vi "RT Main.vi"() -> ()   [LabVIEW 2021]
doc: "Demonstrates the use of the UDP functions to receive broadcast data over a UDP connection."
uses:
  <vilib>/myRIO/Express VI/Onboard Devices/LED/LED Express VI.xnode
  <vilib>/myRIO/Instrument Drivers/Onboard IO/DIO/vis/Write.vi
  <vilib>/myRIO/Instrument Drivers/Onboard IO/DIO/DIO.lvlib
  <vilib>/myRIO/Common/Instrument Driver Framework/myRIO v1.0/DIO/typedefs/DIO Channels Enum.ctl
  <vilib>/myRIO/Common/Instrument Driver Framework/myRIO v1.0/DIO/typedefs/DIO Channels List.ctl
  <vilib>/myRIO/Common/Instrument Driver Framework/Utilities/typedefs/Generic FPGA Reference.ctl
  <vilib>/myRIO/Common/Instrument Driver Framework/Utilities/typedefs/myRIO v1.0 Reference.ctl
  <vilib>/myRIO/Common/Instrument Driver Framework/Utilities/typedefs/Hardware Version Enum.ctl
  <vilib>/myRIO/Common/Instrument Driver Framework/Utilities/typedefs/myRIO Generic Hardware Reference.ctl
  <vilib>/myRIO/Instrument Drivers/Onboard IO/DIO/typedefs/DIO Reference.ctl
  <vilib>/myRIO/Instrument Drivers/Onboard IO/DIO/vis/myRIO DIO Open.xnode
  <vilib>/myRIO/Common/Instrument Driver Framework/Utilities/vis/Is FPGA Ref Available.vi
  <vilib>/myRIO/Instrument Drivers/Utilities/Utilities.lvlib
  <vilib>/myRIO/Common/Instrument Driver Framework/myRIO v1.0/DIO/vis/myRIO v1.1 Open DIO.vi
  <vilib>/userdefined/High Color/nirio_resource_hc.ctl
panel:
  out "error out":errorcluster
  out "LED Status":bool[](array[boolean])
  in  "Stop":bool
  # "Overview: Demonstrates the use of the UDP functions to receive broadcast data over a UDP connection.\nInstructions:\n1. Ensure Desktop Main.vi is already running.\n2. Run this VI.\n3. After you change the value of LED on Desktop Main.vi, observe the value change of LED Status on this VI.\n4. Click Stop to stop this VI."
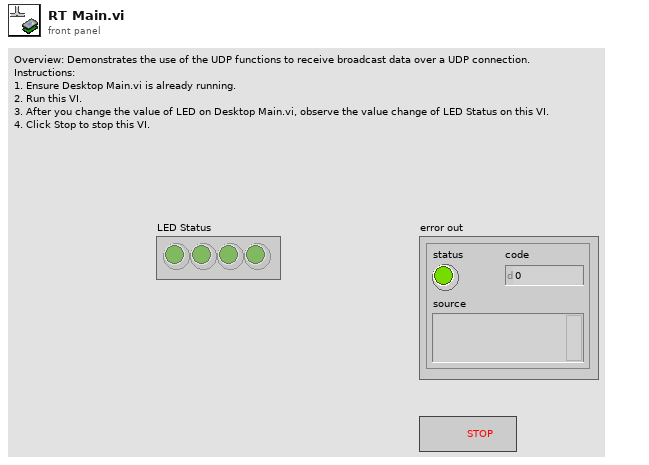
[diagram p1: front panel]
types:
  T1 = typedef "DIO.lvlib/DIO Reference.ctl" = cluster{"myRIO Reference":T2, "DIO Channels List":T6}
  T2 = typedef "myRIO Generic Hardware Reference.ctl" = cluster{"myRIO Model":T3, "myRIO Hardware Reference":T4}
  T3 = typedef "Hardware Version Enum.ctl" = enum16{"Unknown", "myRIO-1900", "myRIO-1950", "roboRIO", "NI ELVIS RIO CM", "ELVIS III"}
  T4 = typedef "myRIO v1.0 Reference.ctl" = cluster{"Generic FPGA Reference":T5, "Allow multiple opens":bool}
  T5 = typedef "Generic FPGA Reference.ctl" = refnum<k20>
  T6 = typedef "DIO Channels List.ctl" = T7[]
  T7 = typedef "DIO Channels Enum.ctl" = enum16{"Not Connected", "C/DIO0", "C/DIO1", "C/DIO2", "C/DIO3", "C/DIO4", "C/DIO5", "C/DIO6", "C/DIO7", "A/DIO0", "A/DIO1", "A/DIO2", "A/DIO3", "A/DIO4", "A/DIO5", "A/DIO6", "A/DIO7", "A/DIO8", "A/DIO9", "A/DIO10", "A/DIO11", "A/DIO12", "A/DIO13", "A/DIO14", "A/DIO15", "A/DIO16", "A/DIO17", "A/DIO18", "A/DIO19", "B/DIO0", "B/DIO1", "B/DIO2", "B/DIO3", "B/DIO4", "B/DIO5", "B/DIO6", "B/DIO7", "B/DIO8", "B/DIO9", "B/DIO10", "B/DIO11", "B/DIO12", "B/DIO13", "B/DIO14", "B/DIO15", "B/DIO16", "B/DIO17", "B/DIO18", "B/DIO19", "LED0", "LED1", "LED2", "LED3", "Button0", "DIO/DIO0", "DIO/DIO1", "DIO/DIO2", "DIO/DIO3", "DIO/DIO4", "DIO/DIO5", "DIO/DIO6", "DIO/DIO7", "DIO/DIO8", "DIO/DIO9", "SPI/CS0", "SPI/CS1", "SPI/CS2", "SPI/CS3", "LED RADIO (Green)", "LED RADIO (Red)", "LED COMM (Green)", "LED COMM (Red)", "LED MODE (Green)", "LED MODE (Red)"}
  T8 = typedef "nirio_resource_hc.ctl" = tag
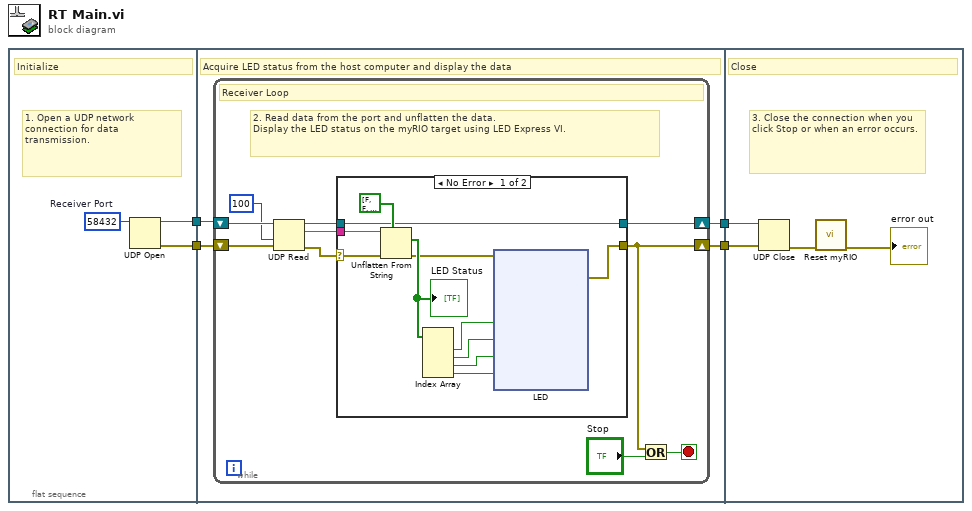
[diagram p0: block diagram]
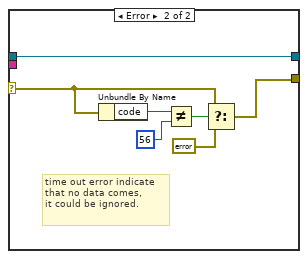
[diagram p2: hidden frame]
diagram:
  n1 = flat-sequence {
    tunnel: [w6] -> w2
    tunnel: [w5] -> w1
    tunnel: [w11] -> w4
    tunnel: [w10] -> w3
    tunnel: w2 -> [w9]
    tunnel: w1 -> [w8]
    tunnel: w4 -> [w80]
    tunnel: w3 -> [w81]
    frame #0 {
      w7 = u16 58432  # Receiver Port
      # "1. Open a UDP network connection for data transmission."
      # "Initialize"
      n2 = UDP Open(11:w7) -> (port=w6:refnum<k16>, 0:w5:errorcluster)  [unwired: 4 in, 1 out]
    }
    frame #1 {
      # "Acquire LED status from the host computer and display the data"
      n3 = while {
        shift-right: [w14] -> w10
        shift-left: w8 -> [w20]
        shift-right: [w12] -> w11
        shift-left: w9 -> [w21]
        stop <- w16 stop-if-true
        # "2. Read data from the port and unflatten the data.\nDisplay the LED status on the myRIO target using LED Express VI."
        # "Receiver Loop"
        n4 = UDP Read(connection ID=w21, timeout ms (25000)=100, 8:w20) -> (data out=w19:string, error out=w15:errorcluster, 3:w13:refnum<k16>)  [unwired: 1 in, 2 out]
        n5 = case shown="No Error" w15 {
          selector: w15 -> [w31 w72]
          tunnel: [w26 w71] -> w14
          tunnel: w19 -> [w32 _]
          tunnel: w13 -> [w28 w77]
          tunnel: [w28 w77] -> w12
          frame No Error {
            n6 = Unflatten From String(type=bool[] [FALSE, FALSE, FALSE, FALSE] ("LED Status"), binary string=w32, error in (no error)=w31) -> (value=w29:bool[], error out=w27:errorcluster)  [unwired: 2 in, 1 out]
            "LED Status" <- w29
            n7 = Index Array(array=w29) -> (element #1=w25:bool, element #2=w24:bool, element #3=w23:bool, element #4=w22:bool)  [unwired: 4 in]
            n8 = xnode "LED"("LED0"=w25, "LED1"=w24, "LED2"=w23, "LED3"=w22, "error in (no error)"=w27) -> ("error out"=w26:errorcluster)
          }
          frame Error {
            # "time out error indicate that no data comes,\nit could be ignored."
            n9 = Unbundle By Name(w72) -> ("code"=w74:i32)
            n10 = Not Equal?(x=w74, y=56) -> (x != y?=w73:bool)
            n11 = Select(t=w72, s=w73, f=errorcluster {"status"=FALSE, "code"=0, "source"=""} ("error out")) -> (s? t:f=w71:errorcluster)
          }
        }
        n12 = Or(x=w14, y="Stop") -> (x .or. y?=w16:bool)
      }
    }
    frame #2 {
      # "3. Close the connection when you click Stop or when an error occurs."
      # "Close"
      n13 = UDP Close(connection ID=w80, 8:w81) -> (error out=w79:errorcluster)  [unwired: 1 out]
      n14 = call <vilib>:"Reset myRIO.vi"("error in (no error)"=w79) -> ("error out"=→"error out":errorcluster)  [unwired: 10 in]
    }
  }
